vi "ma_Spectrum Averaging (real).vi"(3 "real spectrum":dbl[](array[numeric]) format="%0.2f", 4 "df":dbl format="%0.2f", 7 "retrieve last spectrum (F)":bool, 8 "averaging parameters":T1={"averaging mode"=enum."No averaging", "weighting mode"=enum."Exponential", "number of averages"=10} {"number of averages" min=1}, 9 "restart averaging (F)":bool) -> (0 "averaged real spectrum":dbl[](array[numeric]) format="%0.2f", 1 "df":dbl format="%0.2f", 5 "averaging done":bool, 6 "averages completed":dbl format="%0.2f")   [LabVIEW 2020, in "NI_MAPro.lvlib"]
uses:
  NI_MAPro.lvlib
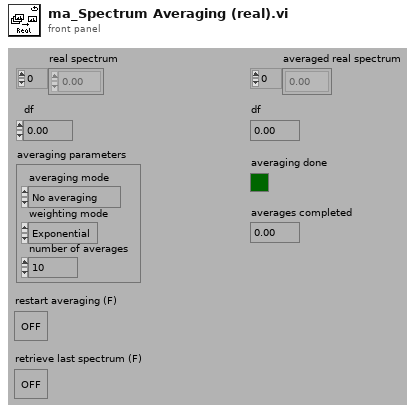
[diagram p1: front panel]
types:
  T1 = cluster{"averaging mode":enum16{"No averaging", "Vector averaging", "RMS averaging", "Peak hold"}, "weighting mode":enum16{"Linear", "Exponential"}, "number of averages":u32}
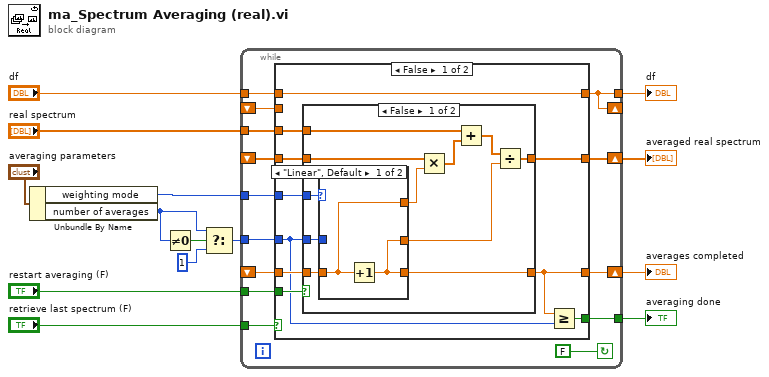
[diagram p0: block diagram]
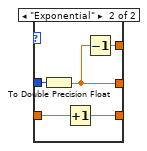
[diagram p2: hidden frame]
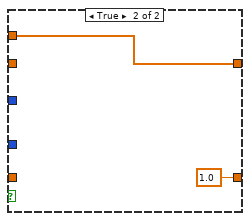
[diagram p3: hidden frame]
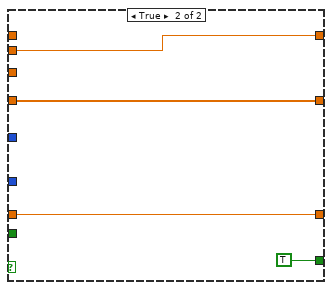
[diagram p4: hidden frame]
diagram:
  n1 = Unbundle By Name("averaging parameters") -> ("weighting mode"=w10:enum16{"Linear", "Exponential"}, "number of averages"=w1:u32)
  n2 = Not Equal To 0?(x=w1) -> (x != 0?=w4:bool)
  n3 = Select(t=w1, s=w4, f=u32 1) -> (s? t:f=w2:u32)
  n4 = while {
    tunnel: [w16] -> w5
    shift-left: _ -> [w15]
    shift-right: [w16] -> _
    tunnel: "df" -> [w17]
    tunnel: "retrieve last spectrum (F)" -> [w19]
    tunnel: [w20] -> w9
    tunnel: w2 -> [w21]
    tunnel: w10 -> [w25]
    tunnel: "real spectrum" -> [w24]
    shift-left: _ -> [w27]
    shift-right: [w22] -> w12
    shift-left: _ -> [w26]
    shift-right: [w28] -> w8
    tunnel: "restart averaging (F)" -> [w23]
    stop <- FALSE continue-if-true
    n5 = case shown="False" w19 {
      tunnel: [w38 w62] -> w28
      tunnel: w27 -> [w37 w61]
      tunnel: w26 -> [w36 w62]
      tunnel: w25 -> [w35 _]
      tunnel: w24 -> [w34 _]
      tunnel: w23 -> [w33 _]
      tunnel: [w32 w61] -> w22
      tunnel: w21 -> [w31 _]
      tunnel: [w30 TRUE] -> w20
      tunnel: w17 -> [w29 _]
      tunnel: [w29 w59] -> w16
      tunnel: w15 -> [_ w59]
      frame False {
        n6 = case shown="False" w33 {
          tunnel: [w46 w57] -> w38
          tunnel: [w41 1.0] -> w32
          tunnel: w37 -> [w44 _]
          tunnel: w36 -> [w49 _]
          tunnel: w34 -> [w45 w57]
          tunnel: w35 -> [w42 _]
          tunnel: w31 -> [w39 _]
          frame False {
            n7 = case shown="\"Linear\", Default" w42 {
              tunnel: w44 -> [w51 w55]
              tunnel: [w50 w56] -> w41
              tunnel: [w51 w52] -> w43
              tunnel: [w50 w53] -> w40
              tunnel: w39 -> [_ w54]
              frame "Linear", Default {
                n8 = Increment(x=w51) -> (x+1=w50:dbl)
              }
              frame "Exponential" {
                n9 = To Double Precision Float(number=w54) -> (double precision float=w53:dbl)
                n10 = Increment(x=w55) -> (x+1=w56:dbl)
                n11 = Decrement(x=w53) -> (x-1=w52:dbl)
              }
            }
            n12 = Multiply(x=w49, y=w43) -> (x*y=w48:dbl[])
            n13 = Add(x=w45, y=w48) -> (x+y=w47:dbl[])
            n14 = Divide(x=w47, y=w40) -> (x/y=w46:dbl[])
          }
          frame True {
          }
        }
        n15 = Greater Or Equal?(x=w32, y=w31) -> (x >= y?=w30:bool)
      }
      frame True {
      }
    }
  }
  "averaged real spectrum" <- w8
  "averages completed" <- w12
  "averaging done" <- w9
  "df" <- w5
